vi "Get Array Elements.vi"(6 "Pass non-arrays":bool, 8 "error in (no error)":errorcluster, 10 "Offset":i32, 11 "JSON":string) -> (0 "error out":errorcluster, 1 "<JSON>":string[](array[string]) caption="<JSON>Elements", 2 "Offset past":i32 caption="Offset past Array")   [LabVIEW 2021, in "json.facade.lvlib"]
doc: "If a JSON Array, returns all elements of the Array.\n\nIf the input JSON is not an Array, this function will return an error, unless \"Pass non-arrays\" is true, in which case the output will be a one-element array containing the input JSON."
uses:
  json.facade.lvlib
  jsontext/JSONtext.lvlib
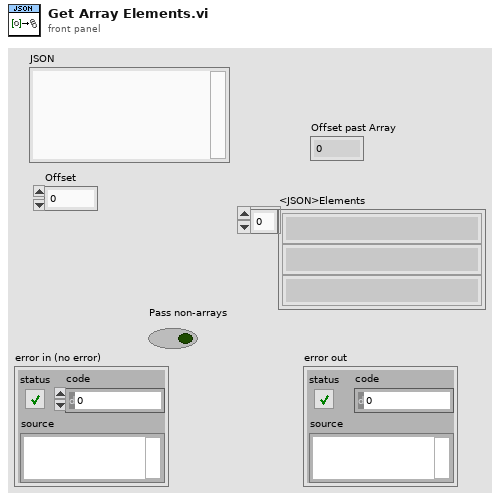
[diagram p1: front panel]
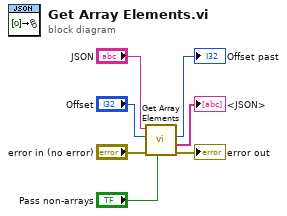
[diagram p0: block diagram]
diagram:
  n1 = call "Get Array Elements.vi"("Pass non-arrays"="Pass non-arrays", "error in (no error)"="error in (no error)", "Offset"="Offset", "JSON"="JSON") -> ("error out"=→"error out":errorcluster, "<JSON>"=→"<JSON>":string[], "Offset past"=→"Offset past":i32)  [unwired: 5 in]
